vi "TestingHumiditySensor.vi"() -> ()   [LabVIEW 2012]
panel:
  out "XY Graph":cluster{"TimeArray":dbl[], "DataArray":dbl[]}[](graph)
  in  "stop":bool
  out "ErrorOut":errorcluster
  out "Data":dbl[](array[numeric])=[26.21, 25.44, 30.22, 15.3]
  in  "Port Number":u16=161
  in  "Write Community String":string="private"
  in  "IP Address":string="192.168.0.170"
  in  "ErrorIn":errorcluster
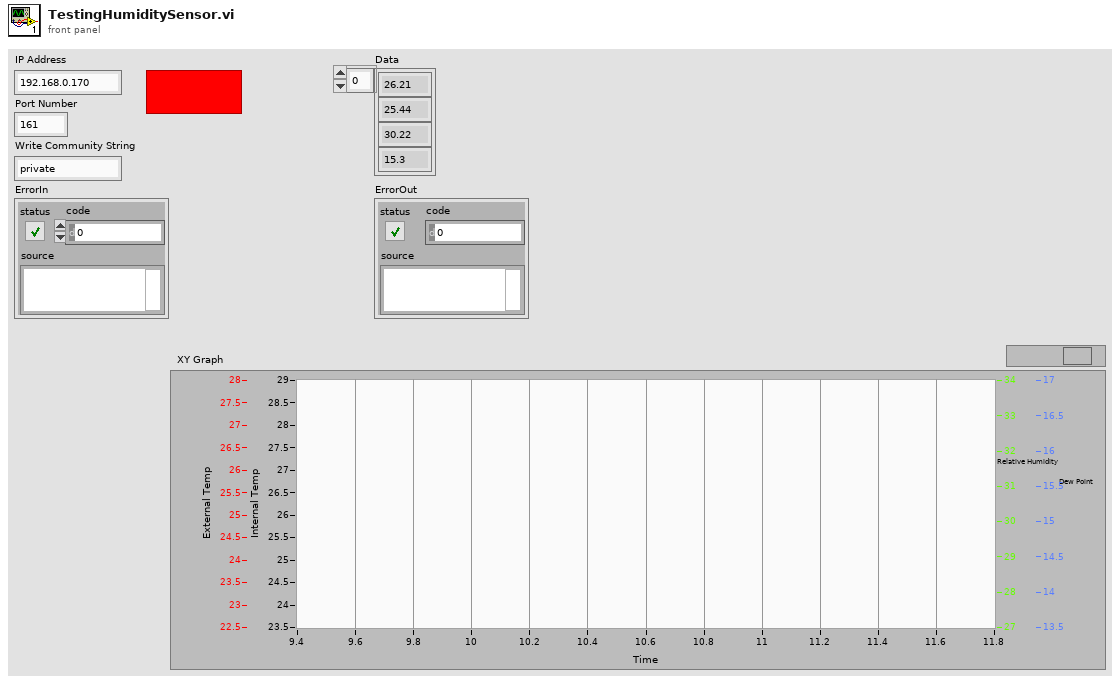
[diagram p1: front panel]
types:
  T1 = cluster{"TimeArrayOut":dbl[], "DataArrayOut":dbl[]}
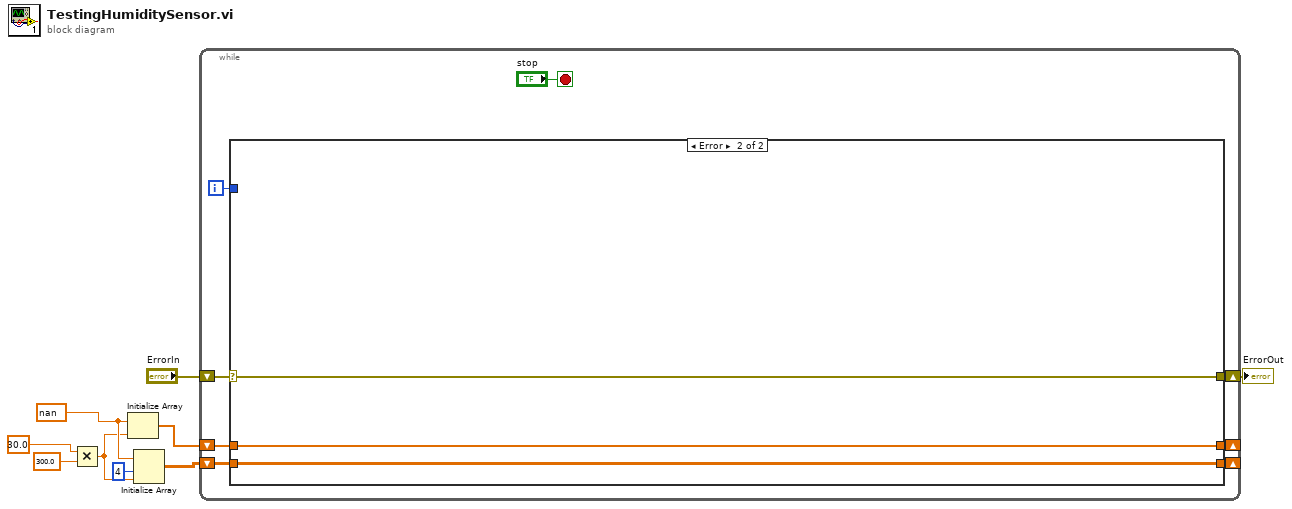
[diagram p0: block diagram]
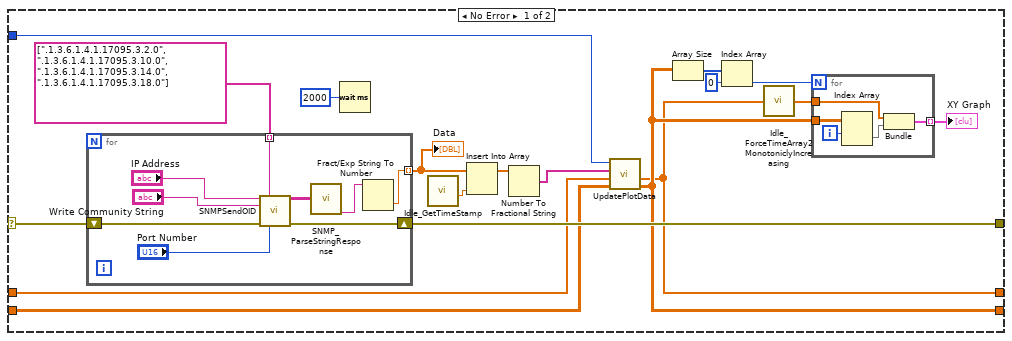
[diagram p2: hidden frame]
diagram:
  w4 = nan ("element")
  n1 = Multiply(x=30.0, y=300.0) -> (x*y=w3:dbl)
  n2 = Initialize Array(w4, w3) -> (w5:dbl[])
  n3 = Initialize Array(w4, 4 ("dimension size"), w3) -> (w1:dbl[][])
  n4 = while {
    shift-right: [w17] -> w8
    shift-left: "ErrorIn" -> [w16]
    shift-right: [w13] -> _
    shift-left: w5 -> [w12]
    shift-right: [w11] -> _
    shift-left: w1 -> [w10]
    i -> [w14]
    stop <- "stop" stop-if-true
    n5 = case shown="Error" w16 {
      selector: w16 -> [w32 w52]
      tunnel: [w33 w52] -> w17
      tunnel: w14 -> [w29 _]
      tunnel: w12 -> [w26 w51]
      tunnel: [w18 w51] -> w13
      tunnel: [w19 w50] -> w11
      tunnel: w10 -> [w25 w50]
      frame No Error {
        n6 = for {
          tunnel: string[] [".1.3.6.1.4.1.17095.3.2.0", ".1.3.6.1.4.1.17095.3.10.0", ".1.3.6.1.4.1.17095.3.14.0", ".1.3.6.1.4.1.17095.3.18.0"] -> [w48] mode=indexing
          shift-right: [w44] -> w33
          shift-left: w32 -> [w49]
          tunnel: [w41] -> w27 mode=indexing
          n7 = call "SNMPSendOID.vi"("IP Address"="IP Address", "OID"=w48, "Write Community String"="Write Community String", "ErrorIn"=w49, "Port Number"="Port Number") -> ("SNMPDataStrings"=w43:string[][], "ErrorOut"=w44:errorcluster)  [unwired: 9 in]
          n8 = call "SNMP_ParseStringResponse.vi"("SNMPDataStrings"=w43) -> ("FirstData"=w42:string)  [unwired: 13 in, 5 out]
          n9 = Fract/Exp String To Number(string=w42) -> (number=w41:dbl)  [unwired: 3 in, 1 out]
        }
        "Data" <- w27
        n10 = Wait (ms)(milliseconds to wait=u32 2000) -> ()  [unwired: 1 out]
        n11 = call "Idle_GetTimeStamp.vi"() -> ("Fractional Hours"=w31:dbl)  [unwired: 11 in]
        n12 = Insert Into Array(array=w27, new element=w31) -> (w30:dbl[])  [unwired: 1 in]
        n13 = Number To Fractional String(number=w30) -> (F-format string=w28:string[])  [unwired: 3 in]
        n14 = call "UpdatePlotData.vi"("DataArrayIn"=w25, "TimeArrayIn"=w26, "DataReturn"=w28, "PlotCount"=w29) -> ("DataArrayOut"=w19:dbl[][], "TimeArrayOut"=w18:dbl[])  [unwired: 6 in]
        n15 = Array Size(array=w19) -> (size(s)=w20:i32[])
        n16 = Index Array(array=w20, index=0) -> (element=w22:i32)
        n17 = call "Idle_ForceTimeArray2MonotoniclyIncreasing.vi"("TimeArrayIn"=w18) -> ("TimeArrayOut"=w24:dbl[])
        n18 = for {
          N: w22 -> [_]
          tunnel: w19 -> [w37]
          tunnel: w24 -> [w36]
          tunnel: [w39] -> w23 mode=indexing
          i -> [w38]
          n19 = Index Array(array=w37, index (row)=w38) -> (element=w40:dbl[])  [unwired: 1 in]
          n20 = Bundle("TimeArrayOut"=w36, "DataArrayOut"=w40) -> (w39:T1)  [unwired: 1 in]
        }
        "XY Graph" <- w23
      }
      frame Error {
      }
    }
  }
  "ErrorOut" <- w8
